vi "Fdx Close Session (Board).vi"(8 "error in (no error)":errorcluster, 11 "InstrumentHandle_board in":u32) -> (0 "error out":errorcluster)   [LabVIEW 2020, in "AIM664LV.lvlib"]
uses:
  AIM664LV.lvlib
  _controls/hwEntry_actions.ctl
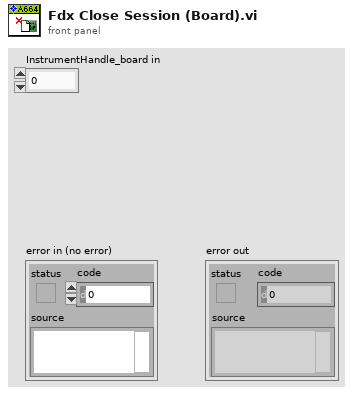
[diagram p1: front panel]
types:
  T1 = typedef "AIM664LV.lvlib/hwEntry_actions.ctl" = enum16{"Init Port", "Init Board", "Relase Port", "Release Board"}
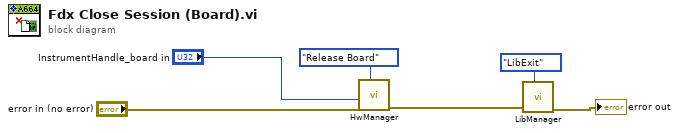
[diagram p0: block diagram]
diagram:
  n1 = call "HwManager.vi"("action (Init)"=hwEntry_actions."Release Board" ("action"), "error in (no error)"="error in (no error)", "InstrumentHandle_board in"="InstrumentHandle_board in") -> ("error out"=w3:errorcluster)  [unwired: 4 in, 4 out]
  n2 = call "LibManager.vi"("action"=enum16{"LibInit", "LibExit"}."LibExit", "error in (no error)"=w3) -> ("error out"=→"error out":errorcluster)  [unwired: 7 in, 2 out]
